vi "Post-Install Custom Action.vi"(10 "Variant":variant) -> (0 "error out":errorcluster)   [LabVIEW 2015]
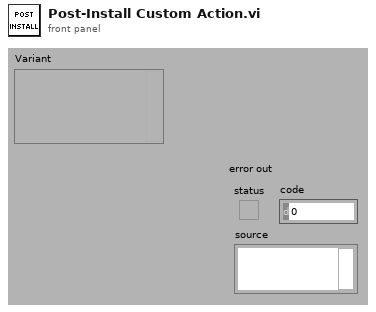
[diagram p1: front panel]
types:
  T1 = typedef "PL_class cache.lvlib/cache definition.ctl" = cluster{"configuration":T2, "class cache data":T3}
  T2 = typedef "PL_class cache.lvlib/cache search configuration.ctl" = cluster{"Search Paths":path[], "Folders to Exclude":string[], "full class list":path[]}
  T3 = typedef "PL_class cache.lvlib/cached class information.ctl" = cluster{"targets":T4[], "engines":T5[], "modules":T5[], "ignored class list":path[]}
  T4 = typedef "PL_class cache.lvlib/target class metadata.ctl" = cluster{"file name":string, "fully qualified name":string, "menu display name":string, "configuration class name":string}
  T5 = typedef "PL_class cache.lvlib/class metadata.ctl" = cluster{"file name":string, "fully qualified name":string, "menu display name":string, "configuration class":string, "category":string, "instances allowed":i32, "supported targets":T6[]}
  T6 = typedef "TBM configuration.lvclass/Target Types.ctl" = enum16{"Windows", "Mac", "Linux", "Linux RT ARM", "VxWorks", "Pharlap", "Other", "Linux RT x64"}
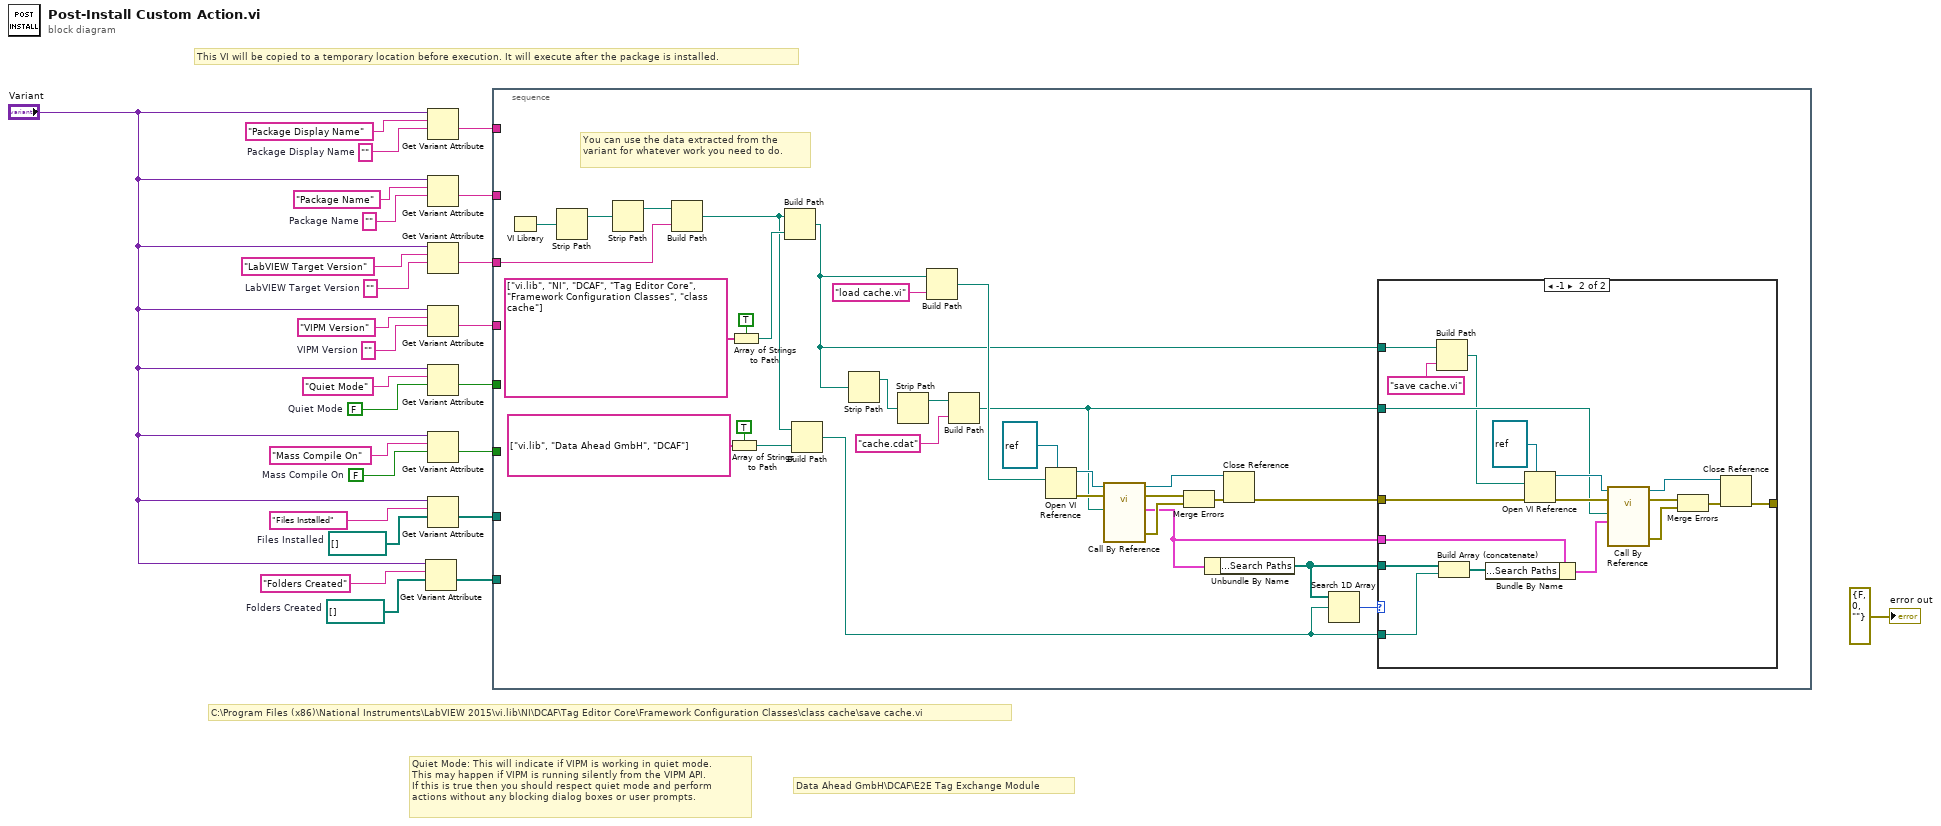
[diagram p0: block diagram]
diagram:
  w1 = path[] []  # Folders Created
  w2 = path[] []  # Files Installed
  w8 = FALSE  # Mass Compile On
  w9 = ""  # Package Display Name
  w16 = FALSE  # Quiet Mode
  w19 = ""  # VIPM Version
  w21 = ""  # LabVIEW Target Version
  w23 = ""  # Package Name
  # "Quiet Mode: This will indicate if VIPM is working in quiet mode.\nThis may happen if VIPM is running silently from the VIPM API.\nIf this is true then you should respect quiet mode and perform\nactions without any blocking dialog boxes or user prompts."
  # "Data Ahead GmbH\\DCAF\\E2E Tag Exchange Module"
  # "C:\\Program Files (x86)\\National Instruments\\LabVIEW 2015\\vi.lib\\NI\\DCAF\\Tag Editor Core\\Framework Configuration Classes\\class cache\\save cache.vi"
  # "This VI will be copied to a temporary location before execution. It will execute after the package is installed."
  n1 = Get Variant Attribute(Variant="Variant", name="Folders Created", default value (empty Variant)=w1) -> (value=w6:path[])  [unwired: 1 in, 3 out]
  n2 = Get Variant Attribute(Variant="Variant", name="Package Display Name", default value (empty Variant)=w9) -> (value=w15:string)  [unwired: 1 in, 3 out]
  n3 = Get Variant Attribute(Variant="Variant", name="Package Name", default value (empty Variant)=w23) -> (value=w14:string)  [unwired: 1 in, 3 out]
  n4 = Get Variant Attribute(Variant="Variant", name="LabVIEW Target Version", default value (empty Variant)=w21) -> (value=w13:string)  [unwired: 1 in, 3 out]
  n5 = Get Variant Attribute(Variant="Variant", name="VIPM Version", default value (empty Variant)=w19) -> (value=w12:string)  [unwired: 1 in, 3 out]
  n6 = Get Variant Attribute(Variant="Variant", name="Quiet Mode", default value (empty Variant)=w16) -> (value=w11:bool)  [unwired: 1 in, 3 out]
  n7 = Get Variant Attribute(Variant="Variant", name="Mass Compile On", default value (empty Variant)=w8) -> (value=w10:bool)  [unwired: 1 in, 3 out]
  n8 = Get Variant Attribute(Variant="Variant", name="Files Installed", default value (empty Variant)=w2) -> (value=w5:path[])  [unwired: 1 in, 3 out]
  n9 = stacked-sequence {
    tunnel: w15 -> [_]
    tunnel: w14 -> [_]
    tunnel: w13 -> [w53]
    tunnel: w12 -> [_]
    tunnel: w11 -> [_]
    tunnel: w10 -> [_]
    tunnel: w5 -> [_]
    tunnel: w6 -> [_]
    frame #0 {
      # "You can use the data extracted from the variant for whatever work you need to do."
      n10 = VI Library() -> (path=w56:path)
      n11 = Strip Path(path=w56) -> (stripped path=w55:path)  [unwired: 1 out]
      n12 = Strip Path(path=w55) -> (stripped path=w54:path)  [unwired: 1 out]
      n13 = Build Path(base path=w54, name or relative path=w53) -> (appended path=w29:path)
      n14 = Array of Strings to Path(0:string[] ["vi.lib", "Data Ahead GmbH", "DCAF"], 1:TRUE ("relative")) -> (2:w28:path)
      n15 = Array of Strings to Path(0:string[] ["vi.lib", "NI", "DCAF", "Tag Editor Core", "Framework Configuration Classes", "class cache"], 1:TRUE ("relative")) -> (2:w50:path)
      n16 = Build Path(base path=w29, name or relative path=w50) -> (appended path=w32:path)
      n17 = Build Path(base path=w29, name or relative path=w28) -> (appended path=w27:path)
      n18 = Strip Path(path=w32) -> (stripped path=w44:path)  [unwired: 1 out]
      n19 = Strip Path(path=w44) -> (stripped path=w43:path)  [unwired: 1 out]
      n20 = Build Path(base path=w32, name or relative path="load cache.vi") -> (appended path=w47:path)
      n21 = Build Path(base path=w43, name or relative path="cache.cdat") -> (appended path=w33:path)
      n22 = Open VI Reference(type specifier VI Refnum (for type only)=refnum<vi> refnum, vi path=w47) -> (vi reference=w45:refnum<vi>, error out=w46:errorcluster)  [unwired: 4 in]
      n23 = call-by-ref "?"(reference=w45, error in=w46, "cache path"=w33) -> (reference out=w38:refnum<vi>, error out=w41:errorcluster, 0:"error out"=w40:errorcluster, "cache"=w35:T1)  [unwired: 9 in]
      n24 = Merge Errors(w41, w40) -> (w39:errorcluster)
      n25 = Unbundle By Name(w35) -> ("configuration.Search Paths"=w36:path[])
      n26 = Close Reference(reference=w38, error in (no error)=w39) -> (error out=w34:errorcluster)
      n27 = Search 1D Array(1D array=w36, element=w27) -> (index of element=w37:i32)  [unwired: 1 in]
      n28 = case shown="-1" w37 {
        tunnel: w36 -> [_ w75]
        tunnel: w35 -> [_ w73]
        tunnel: w34 -> [w57 w71]
        tunnel: w33 -> [_ w67]
        tunnel: w32 -> [_ w65]
        tunnel: w27 -> [_ w59]
        tunnel: [w57 w58] -> _
        frame Default {
        }
        frame -1 {
          n29 = Build Path(base path=w65, name or relative path="save cache.vi") -> (appended path=w64:path)
          n30 = Build Array (concatenate)(w75, w59) -> (w74:path[])
          n31 = Bundle By Name(cluster=w73, "configuration.Search Paths"=w74) -> (w68:T1)
          n32 = Open VI Reference(type specifier VI Refnum (for type only)=refnum<vi> refnum, vi path=w64, error in (no error)=w71) -> (vi reference=w69:refnum<vi>, error out=w70:errorcluster)  [unwired: 3 in]
          n33 = call-by-ref "?"(reference=w69, error in=w70, "cache"=w68, "path"=w67) -> (reference out=w60:refnum<vi>, error out=w63:errorcluster, 0:"error out"=w62:errorcluster)  [unwired: 9 in]
          n34 = Merge Errors(w63, w62) -> (w61:errorcluster)
          n35 = Close Reference(reference=w60, error in (no error)=w61) -> (error out=w58:errorcluster)
        }
      }
    }
  }
  "error out" <- errorcluster {"status"=FALSE, "code"=0, "source"=""} ("error out")
